vi "bus_monitor_server_api.StartServer.vi"(8 "error in (no error)":errorcluster, 11 "gRPC Container in":refnum<class "bus_monitor_server_api.lvclass">) -> (0 "error out":errorcluster, 3 "gRPC Container out":refnum<class "bus_monitor_server_api.lvclass">)   [LabVIEW 2025, in "bus_monitor_server_api.lvlib" / "bus_monitor_server_api.lvclass"]
uses:
  bus_monitor_server_api.lvclass
  bus_monitor_server_api.lvclass/bus_monitor_server_api.ctl
  <vilib>/Utility/SystemLogging/NI_SystemLogging.lvlib
  bus_monitor_server/bus_monitor_server.lvlib
  <vilib>/gRPC/LabVIEW gRPC Servicer/Servicer/Servicer.lvclass
  <vilib>/gRPC/LabVIEW gRPC Servicer/ServiceBase/ServiceBase.lvclass
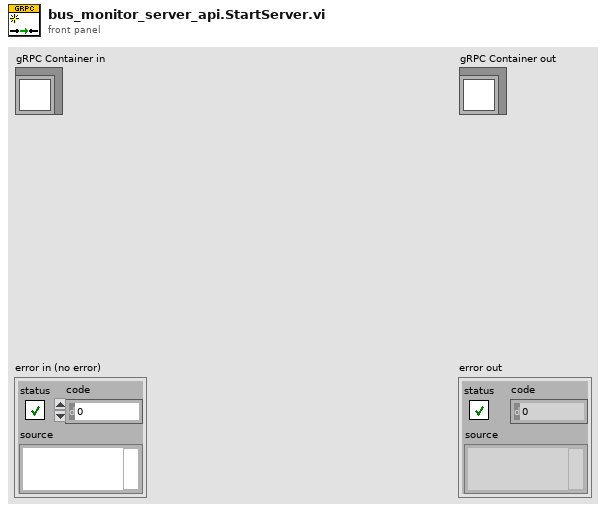
[diagram p1: front panel]
types:
  T1 = typedef "grpc-lvsupport-release.lvlib/grpcId.ctl" = u64
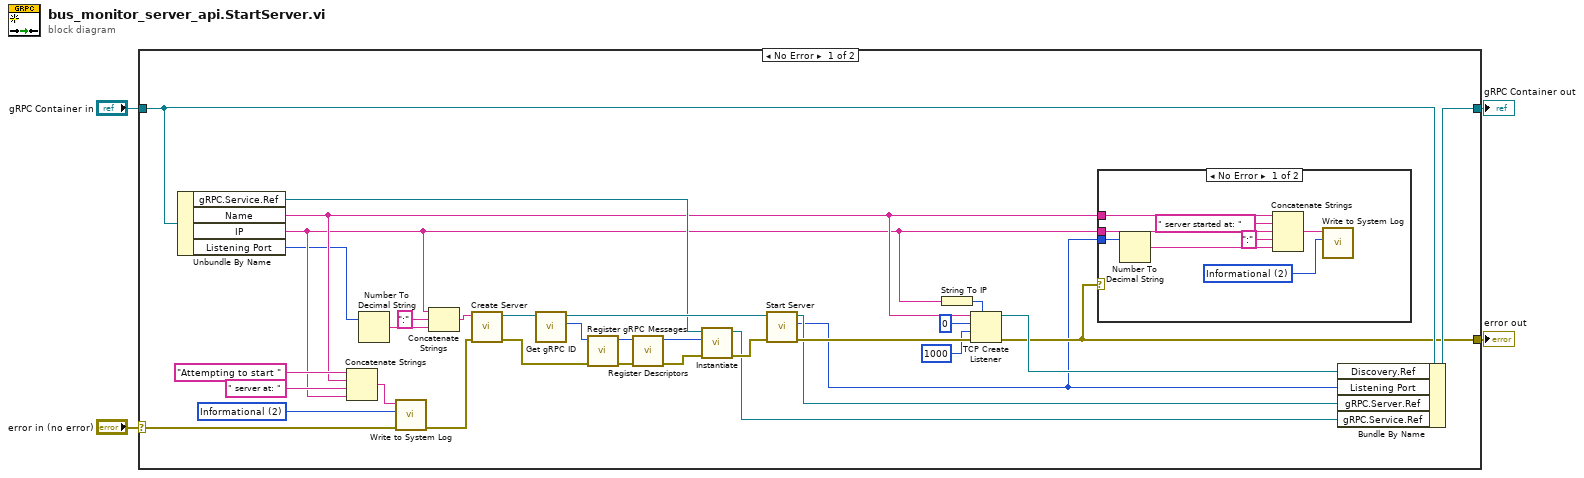
[diagram p0: block diagram]
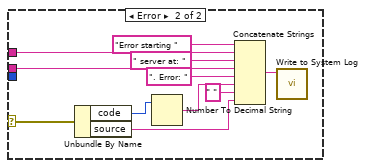
[diagram p2: hidden frame]
diagram:
  n1 = case shown="No Error" "error in (no error)" {
    selector: "error in (no error)" -> [w23 w58]
    tunnel: [w13 w58] -> w3
    tunnel: [w24 w57] -> w1
    tunnel: "gRPC Container in" -> [w25 w57]
    frame No Error {
      w27 = 2 items=["Error", "Warning", "Informational"] ("severity")
      n2 = Unbundle By Name(w25) -> ("gRPC.Service.Ref"=w19:refnum<class "ServiceBase.lvclass">, "Name"=w16:string, "IP"=w15:string, "Listening Port"=w9:i32)
      n3 = Concatenate Strings("Attempting to start " ("string"), w16, " server at: " ("string"), w15) -> (w26:string)
      n4 = Number To Decimal String(number=w9) -> (decimal integer string=w10:string)  [unwired: 1 in]
      n5 = call <vilib>:"Write to System Log.vi"("error in (no error)"=w23, "severity"=w27, "message"=w26) -> ("error out"=w11:errorcluster)  [unwired: 8 in]
      n6 = Concatenate Strings(w15, ":" ("string"), w10) -> (w20:string)
      n7 = call <vilib>:"Create Server.vi"("error in"=w11, "Server Address"=w20) -> ("error out"=w32:errorcluster, "gRPC server out"=w31:refnum<class "Servicer.lvclass">)  [unwired: 8 in]
      n8 = call <vilib>:"Get gRPC ID.vi"("gRPC server in"=w31) -> ("gRPC ID"=w37:T1, "gRPC server out"=w30:refnum<class "Servicer.lvclass">)  [unwired: 9 in]
      n9 = call "Register gRPC Messages.vi"("error in (no error)"=w32, "gRPC ID"=w37) -> ("error out"=w36:errorcluster, "gRPC ID Out"=w35:T1)  [unwired: 8 in]
      n10 = call "Register Descriptors.vi"("error in (no error)"=w36, "gRPC ID"=w35) -> ("error out"=w34:errorcluster, "gRPC ID Out"=w33:T1)  [unwired: 8 in]
      n11 = call-dynamic "Instantiate.vi"("error in"=w34, "gRPCid"=w33, "gRPC service in"=w19) -> ("error out"=w28:errorcluster, "gRPC service out"=w18:refnum<class "ServiceBase.lvclass">)  [unwired: 7 in]
      n12 = call <vilib>:"Start Server.vi"("error in"=w28, "gRPC server in"=w30) -> ("error out"=w14:errorcluster, "Listening Port"=w8:i32, "gRPC server out"=w12:refnum<class "Servicer.lvclass">)  [unwired: 7 in]
      n13 = String To IP(1:w15) -> (0:w5:u32)
      n14 = TCP Create Listener(7:w5, 8:w14, 9:1000 ("timeout ms (25000)"), 10:u16 0 ("port"), 11:w16) -> (0:w13:errorcluster, 3:w17:refnum<k5>)  [unwired: 1 out]
      n15 = case shown="No Error" w13 {
        selector: w13 -> [_ w49]
        tunnel: w16 -> [w42 w48]
        tunnel: w15 -> [w40 w46]
        tunnel: w8 -> [w41 _]
        frame No Error {
          w43 = 2 items=["Error", "Warning", "Informational"] ("severity")
          n16 = Number To Decimal String(number=w41) -> (decimal integer string=w38:string)  [unwired: 1 in]
          n17 = Concatenate Strings(w42, " server started at: " ("string"), w40, ":" ("string"), w38) -> (w45:string)
          n18 = call <vilib>:"Write to System Log.vi"("severity"=w43, "message"=w45) -> ()  [unwired: 9 in, 1 out]
        }
        frame Error {
          n19 = Unbundle By Name(w49) -> ("code"=w53:i32, "source"=w54:string)
          n20 = Number To Decimal String(number=w53) -> (decimal integer string=w52:string)  [unwired: 1 in]
          n21 = Concatenate Strings("Error starting " ("string"), w48, " server at: " ("string"), w46, ". Error: " ("string"), w52, " " ("string"), w54) -> (w50:string)
          n22 = call <vilib>:"Write to System Log.vi"("message"=w50) -> ()  [unwired: 10 in, 1 out]
        }
      }
      n23 = Bundle By Name(cluster=w25, "Discovery.Ref"=w17, "Listening Port"=w8, "gRPC.Server.Ref"=w12, "gRPC.Service.Ref"=w18) -> (w24:refnum<class "bus_monitor_server_api.lvclass">)
    }
    frame Error {
    }
  }
  "error out" <- w3
  "gRPC Container out" <- w1
